vi "ep_Flicker Cumulative Probability Function.vi"(0 "instantaneous flicker Pinst (Output 5)":waveform(dbl), 1 "restart (F)":bool) -> (4 "flicker cumulative probability function":dbl[](array[numeric]), 6 "Pst flicker time":timestamp, 15 "data valid?":bool)   [LabVIEW 2011, in "NI_EP_Power Quality.lvlib"]
uses:
  <vilib>/addons/Electrical Power/PQ/NI_EP_Power Quality.lvlib
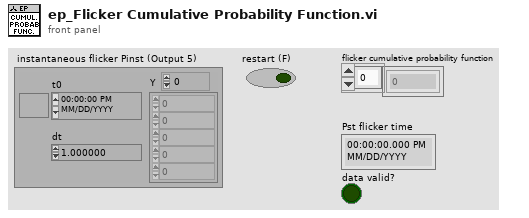
[diagram p1: front panel]
types:
  T1 = typedef "LVDateTimeRec.ctl" = cluster{"fractional second":dbl, "second":i32, "minute":i32, "hour":i32, "day of month":i32, "month":i32, "year":i32, "day of week":i32, "day of year":i32, "DST":i32}
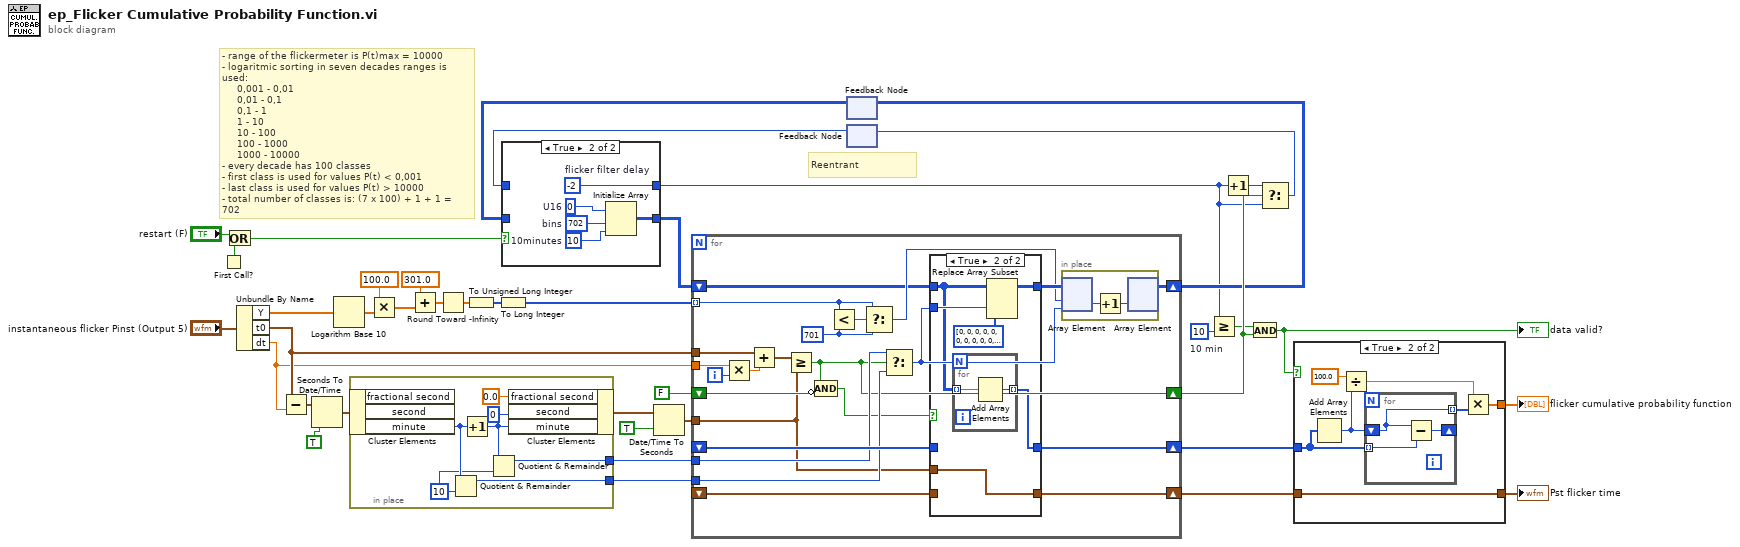
[diagram p0: block diagram]
diagram:
  w14 = 10  # 10 min
  # "- range of the flickermeter is P(t)max = 10000\n- logaritmic sorting in seven decades ranges is used:\n     0,001 - 0,01\n     0,01 - 0,1\n     0,1 - 1\n     1 - 10\n     10 - 100 \n     100 - 1000\n     1000 - 10000\n- every decade has 100 classes\n- first class is used for values P(t) < 0,001\n- last class is used for values P(t) > 10000\n- total number of classes is: (7 x 100) + 1 + 1 = 702"
  # "Reentrant"
  n1 = First Call?() -> (First Call?: T/F=w24:bool)
  n2 = Or(x="restart (F)", y=w24) -> (x .or. y?=w36:bool)
  n3 = Unbundle By Name("instantaneous flicker Pinst (Output 5)") -> ("Y"=w34:dbl[], "t0"=w39:timestamp, "dt"=w37:dbl)
  n4 = Subtract(x=w39, y=w37) -> (x-y=w38:timestamp)
  n5 = Seconds To Date/Time(time stamp (now)=w38, to UTC (F)=TRUE) -> (date time rec=w26:T1)
  n6 = Logarithm Base 10(1:w34) -> (0:w5:dbl[])
  n7 = in-place {
    in-place-border: [w43] -> w29
    in-place-border: [w41] -> w30
    w40 = 10 ("y")
    n8 = in-place-cluster #1(w26) -> ("minute"=w44:i32)  [unwired: 2 out]
    n9 = Quotient & Remainder(x=w44, y=w40) -> (x-y*floor(x/y)=w43:i32)  [unwired: 1 out]
    n10 = Increment(x=w44) -> (x+1=w42:i32)
    n11 = Quotient & Remainder(x=w42, y=w40) -> (x-y*floor(x/y)=w41:i32)  [unwired: 1 out]
    n12 = in-place-cluster #1("fractional second"=0.0, "second"=0, "minute"=w42) -> (w31:T1)
  }
  n13 = Multiply(x=100.0, y=w5) -> (x*y=w1:dbl[])
  n14 = Add(x=301.0, y=w1) -> (x+y=w3:dbl[])
  n15 = Round Toward -Infinity(1:w3) -> (0:w7:dbl[])
  n16 = To Unsigned Long Integer(number=w7) -> (unsigned 32bit integer=w6:u32[])
  n17 = To Long Integer(number=w6) -> (32bit integer=w35:i32[])
  n18 = Date/Time To Seconds(1:TRUE ("is UTC (F)"), 2:w31) -> (0:w32:timestamp)
  n19 = feedback #2() -> (w10:u16[][])  [unwired: 1 in]
  n20 = feedback #3() -> (w13:i32)  [unwired: 1 in]
  n21 = case shown="True" w36 {
    tunnel: [w48 w50] -> w11
    tunnel: w10 -> [w48 _]
    tunnel: [w47 w49] -> w18
    tunnel: w13 -> [w47 _]
    frame False {
    }
    frame True {
      w49 = -2  # flicker filter delay
      w51 = 10  # 10minutes
      w52 = 702  # bins
      w53 = u16 0  # U16
      n22 = Initialize Array(w53, w52, w51) -> (w50:u16[][])
    }
  }
  n23 = for {
    shift-right: [w75] -> w23
    shift-left: w11 -> [w70]
    tunnel: w35 -> [w74] mode=indexing
    shift-right: [w65] -> w20
    shift-left: _ -> [w64]
    tunnel: w37 -> [w68]
    tunnel: w39 -> [w67]
    shift-right: [w63] -> w16
    shift-left: _ -> [w62]
    shift-right: [w57] -> w33
    shift-left: FALSE -> [w61]
    tunnel: w29 -> [w60]
    tunnel: w30 -> [w59]
    tunnel: w32 -> [w56]
    i -> [w66]
    w73 = 701 ("y")
    n24 = Multiply(x=w68, y=w66) -> (x*y=w69:dbl)
    n25 = Add(x=w67, y=w69) -> (x+y=w54:timestamp)
    n26 = Greater Or Equal?(x=w54, y=w56) -> (x >= y?=w57:bool)
    n27 = Compound Arithmetic op=AND(w57, invert w61) -> (w55:bool)
    n28 = Less?(x=w74, y=w73) -> (x < y?=w76:bool)
    n29 = Select(t=w74, s=w76, f=w73) -> (s? t:f=w71:i32)
    n30 = Select(t=w59, s=w57, f=w60) -> (s? t:f=w58:i32)
    n31 = case shown="True" w55 {
      tunnel: w70 -> [w79 w82]
      tunnel: [w79 w85] -> w72
      tunnel: w58 -> [_ w84]
      tunnel: [w78 w81] -> w65
      tunnel: w64 -> [w78 _]
      tunnel: [w77 w80] -> w63
      tunnel: w62 -> [w77 _]
      tunnel: w56 -> [_ w80]
      frame False {
      }
      frame True {
        n32 = for {
          tunnel: w82 -> [w87] mode=indexing
          tunnel: [w86] -> w81 mode=indexing
          n33 = Add Array Elements(numeric array=w87) -> (sum=w86:u16)
        }
        n34 = Replace Array Subset(array=w82, new element=u16[] [0, 0, 0, 0, 0, 0, 0, 0, 0, 0, 0, 0, 0, 0, 0, 0, 0, 0, 0, 0, 0, 0, 0, 0, 0, 0, 0, 0, 0, 0, 0, 0, 0, 0, 0, 0, 0, 0, 0, 0, 0, 0, 0, 0, 0, 0, 0, 0, 0, 0, 0, 0, 0, 0, 0, 0, 0, 0, 0, 0, 0, 0, 0, 0, 0, 0, 0, 0, 0, 0, 0, 0, 0, 0, 0, 0, 0, 0, 0, 0, 0, 0, 0, 0, 0, 0, 0, 0, 0, 0, 0, 0, 0, 0, 0, 0, 0, 0, 0, 0, 0, 0, 0, 0, 0, 0, 0, 0, 0, 0, 0, 0, 0, 0, 0, 0, 0, 0, 0, 0, 0, 0, 0, 0, 0, 0, 0, 0, 0, 0, 0, 0, 0, 0, 0, 0, 0, 0, 0, 0, 0, 0, 0, 0, 0, 0, 0, 0, 0, 0, 0, 0, 0, 0, 0, 0, 0, 0, 0, 0, 0, 0, 0, 0, 0, 0, 0, 0, 0, 0, 0, 0, 0, 0, 0, 0, 0, 0, 0, 0, 0, 0, 0, 0, 0, 0, 0, 0, 0, 0, 0, 0, 0, 0, 0, 0, 0, 0, 0, 0, 0, 0, 0, 0, 0, 0, 0, 0, 0, 0, 0, 0, 0, 0, 0, 0, 0, 0, 0, 0, 0, 0, 0, 0, 0, 0, 0, 0, 0, 0, 0, 0, 0, 0, 0, 0, 0, 0, 0, 0, 0, 0, 0, 0, 0, 0, 0, 0, 0, 0, 0, 0, 0, 0, 0, 0, 0, 0, 0, 0, 0, 0, 0, 0, 0, 0, 0, 0, 0, 0, 0, 0, 0, 0, 0, 0, 0, 0, 0, 0, 0, 0, 0, 0, 0, 0, 0, 0, 0, 0, 0, 0, 0, 0, 0, 0, 0, 0, 0, 0, 0, 0, 0, 0, 0, 0, 0, 0, 0, 0, 0, 0, 0, 0, 0, 0, 0, 0, 0, 0, 0, 0, 0, 0, 0, 0, 0, 0, 0, 0, 0, 0, 0, 0, 0, 0, 0, 0, 0, 0, 0, 0, 0, 0, 0, 0, 0, 0, 0, 0, 0, 0, 0, 0, 0, 0, 0, 0, 0, 0, 0, 0, 0, 0, 0, 0, 0, 0, 0, 0, 0, 0, 0, 0, 0, 0, 0, 0, 0, 0, 0, 0, 0, 0, 0, 0, 0, 0, 0, 0, 0, 0, 0, 0, 0, 0, 0, 0, 0, 0, 0, 0, 0, 0, 0, 0, 0, 0, 0, 0, 0, 0, 0, 0, 0, 0, 0, 0, 0, 0, 0, 0, 0, 0, 0, 0, 0, 0, 0, 0, 0, 0, 0, 0, 0, 0, 0, 0, 0, 0, 0, 0, 0, 0, 0, 0, 0, 0, 0, 0, 0, 0, 0, 0, 0, 0, 0, 0, 0, 0, 0, 0, 0, 0, 0, 0, 0, 0, 0, 0, 0, 0, 0, 0, 0, 0, 0, 0, 0, 0, 0, 0, 0, 0, 0, 0, 0, 0, 0, 0, 0, 0, 0, 0, 0, 0, 0, 0, 0, 0, 0, 0, 0, 0, 0, 0, 0, 0, 0, 0, 0, 0, 0, 0, 0, 0, 0, 0, 0, 0, 0, 0, 0, 0, 0, 0, 0, 0, 0, 0, 0, 0, 0, 0, 0, 0, 0, 0, 0, 0, 0, 0, 0, 0, 0, 0, 0, 0, 0, 0, 0, 0, 0, 0, 0, 0, 0, 0, 0, 0, 0, 0, 0, 0, 0, 0, 0, 0, 0, 0, 0, 0, 0, 0, 0, 0, 0, 0, 0, 0, 0, 0, 0, 0, 0, 0, 0, 0, 0, 0, 0, 0, 0, 0, 0, 0, 0, 0, 0, 0, 0, 0, 0, 0, 0, 0, 0, 0, 0, 0, 0, 0, 0, 0, 0, 0, 0, 0, 0, 0, 0, 0, 0, 0, 0, 0, 0, 0, 0, 0, 0, 0, 0, 0, 0, 0, 0, 0, 0, 0, 0, 0, 0, 0, 0, 0, 0, 0, 0, 0, 0, 0, 0, 0, 0, 0, 0, 0, 0, 0, 0, 0, 0, 0, 0, 0, 0, 0, 0, 0, 0, 0, 0, 0, 0, 0, 0, 0, 0, 0, 0, 0, 0, 0, 0, 0, 0, 0, 0, 0, 0, 0, 0, 0, 0, 0, 0, 0, 0, 0, 0, 0] ("x*y"), index (col)=w84) -> (w85:u16[][])  [unwired: 1 in]
      }
    }
    n35 = in-place {
      n36 = in-place-array #4(w72, w71, w58) -> (w89:u16)
      n37 = Increment(x=w89) -> (x+1=w88:u16)
      n38 = in-place-array #4(w88) -> (w75:u16[][])  [unwired: 2 out]
    }
  }
  n39 = feedback-in #2(w23) -> ()
  n40 = Greater Or Equal?(x=w18, y=w14) -> (x >= y?=w15:bool)
  n41 = Increment(x=w18) -> (x+1=w12:i32)
  n42 = And(x=w15, y=w33) -> (x .and. y?=w21:bool)
  "data valid?" <- w21
  n43 = Select(t=w12, s=w33, f=w18) -> (s? t:f=w22:i32)
  n44 = feedback-in #3(w22) -> ()
  n45 = case shown="True" w21 {
    tunnel: w16 -> [_ w95]
    tunnel: [_ w95] -> w17
    tunnel: [_ w92] -> w19
    tunnel: w20 -> [_ w96]
    frame False {
    }
    frame True {
      n46 = Add Array Elements(numeric array=w96) -> (sum=w93:u16)
      n47 = Divide(x=100.0, y=w93) -> (x/y=w90:dbl)
      n48 = for {
        tunnel: w96 -> [w97] mode=indexing
        shift-right: [w99] -> _
        shift-left: w93 -> [w98]
        tunnel: [w98] -> w91 mode=indexing
        n49 = Subtract(x=w98, y=w97) -> (x-y=w99:u16)
      }
      n50 = Multiply(x=w90, y=w91) -> (x*y=w92:dbl[])
    }
  }
  "flicker cumulative probability function" <- w19
  "Pst flicker time" <- w17
